vi "AddNewChat.vi"(10 "result":T1, 11 "ActiveChats in":cluster{"ChatId":i32, "Type":string}[](array[cluster])) -> (3 "ActiveChats out":cluster{"ChatId":i32, "Type":string}[](array[cluster]))   [LabVIEW 2015]
uses:
  Telegram/Methods/TypeDefs/UpdateUniversal.ctl
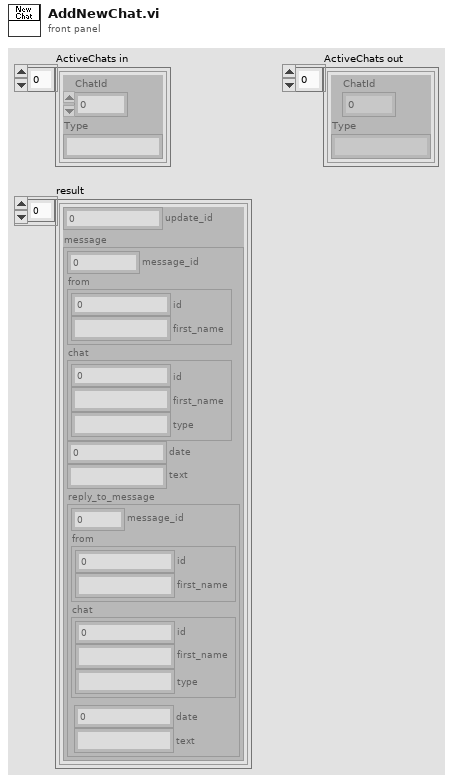
[diagram p1: front panel]
types:
  T1 = typedef "UpdateUniversal.ctl" = cluster{"update_id":u32, "message":cluster{"message_id":u32, "from":cluster{"id":u32, "first_name":string}, "chat":cluster{"id":i32, "first_name":string, "type":string}, "date":u32, "text":string, "reply_to_message":cluster{"message_id":u32, "from":cluster{"id":u32, "first_name":string}, "chat":cluster{"id":i32, "first_name":string, "type":string}, "date":u32, "text":string}}}[]
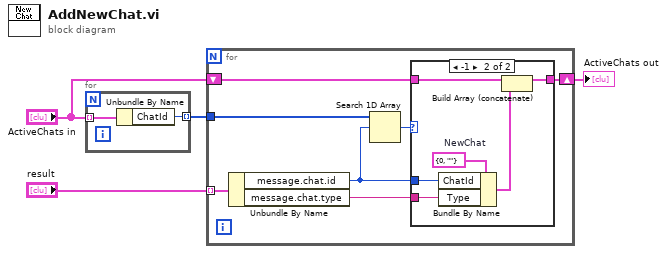
[diagram p0: block diagram]
diagram:
  n1 = for {
    tunnel: "ActiveChats in" -> [w6] mode=indexing
    tunnel: [w5] -> w1 mode=indexing
    n2 = Unbundle By Name(w6) -> ("ChatId"=w5:i32)
  }
  n3 = for {
    tunnel: w1 -> [w13]
    shift-right: [w10] -> w4
    shift-left: "ActiveChats in" -> [w11]
    tunnel: "result" -> [w9] mode=indexing
    n4 = Unbundle By Name(w9) -> ("message.chat.id"=w7:i32, "message.chat.type"=w8:string)
    n5 = Search 1D Array(1D array=w13, element=w7) -> (index of element=w12:i32)  [unwired: 1 in]
    n6 = case shown="-1" w12 {
      tunnel: w11 -> [w14 w17]
      tunnel: [w14 w15] -> w10
      tunnel: w7 -> [_ w18]
      tunnel: w8 -> [_ w19]
      frame Default {
      }
      frame -1 {
        w20 = cluster{"ChatId":i32, "Type":string} {"ChatId"=0, "Type"=""}  # NewChat
        n7 = Bundle By Name(cluster=w20, "ChatId"=w18, "Type"=w19) -> (w16:cluster{"ChatId":i32, "Type":string})
        n8 = Build Array (concatenate)(w17, w16) -> (w15:cluster{"ChatId":i32, "Type":string}[])
      }
    }
  }
  "ActiveChats out" <- w4
